vi "DHE_SetSampling.vi"(7 "DBS Ref":T1, 8 "error in":errorcluster, 10 "sampling type":string, 11 "fd":i32) -> (0 "error out":errorcluster, 2 "read value":i32, 3 "fd":i32)   [LabVIEW 2016]
uses:
  DBSHAND/private/vis/DatabaseHand_RefNum.ctl
  DBSHAND/private/vis/DatabaseHand_Element_Set(bool).vi
  DBSHAND/private/vis/DatabaseHand_Element_Set(string).vi
  DBSHAND/private/vis/DatabaseHand_Element_Get(string).vi
  DBSHAND/private/vis/DatabaseHand_Element_Set(I32).vi
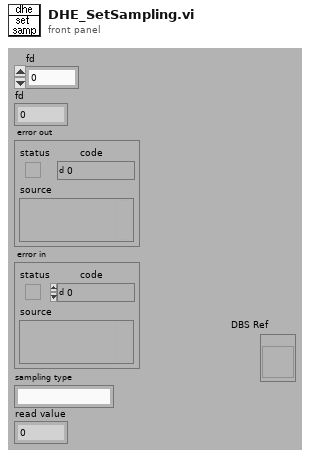
[diagram p1: front panel]
types:
  T1 = typedef "DatabaseHand_RefNum.ctl" = refnum<vi>
  T2 = cluster{"Video Processor Type":string, "support gain":bool, "Timing Board":string, "support reset":bool, "Utility Board":string, "Shutter":string, "Temperature":string, "support temp control":bool, "Detector Type":string, "Support MPP":string, "Support Binning":string, "Readout Mode":string, "support shutter control":bool}
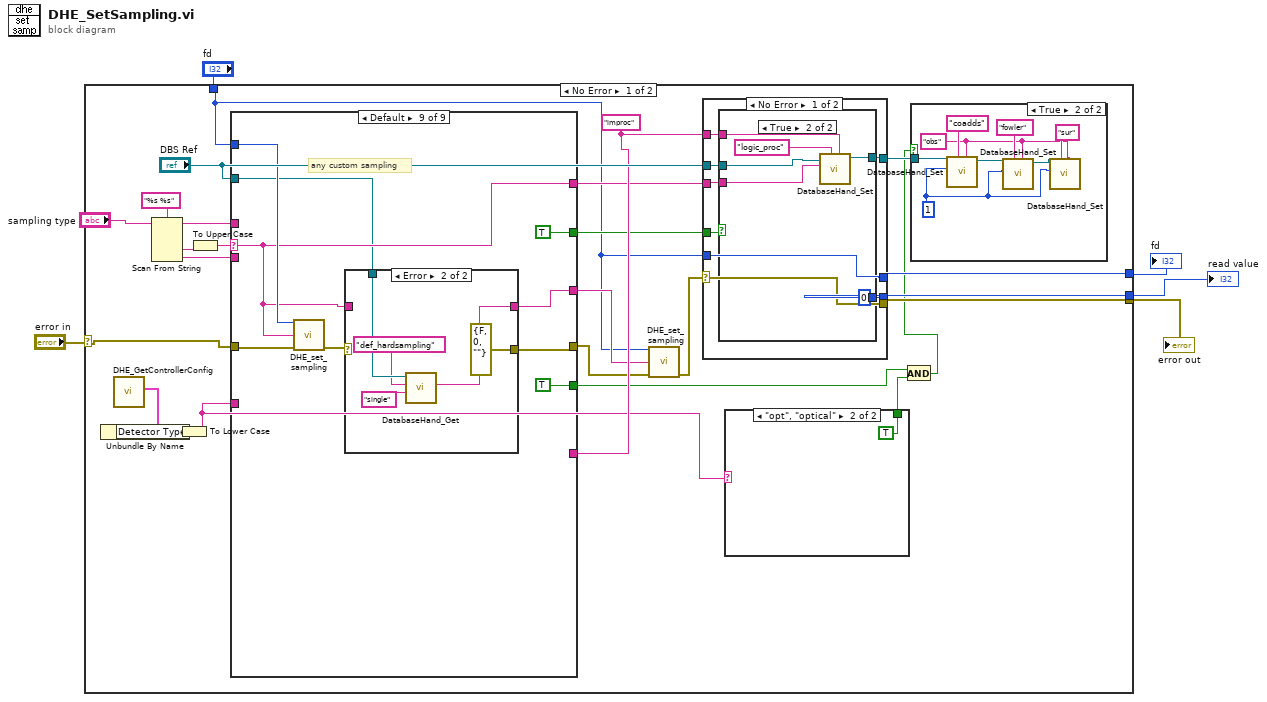
[diagram p0: block diagram]
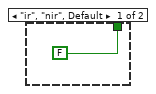
[diagram p2: hidden frame]
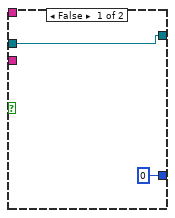
[diagram p4: hidden frame]
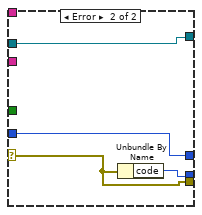
[diagram p5: hidden frame]
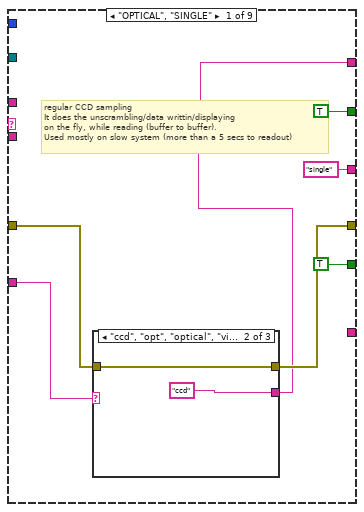
[diagram p6: hidden frame]
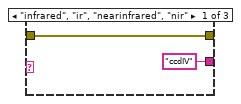
[diagram p7: hidden frame]
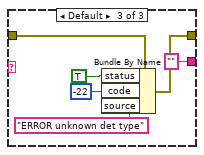
[diagram p8: hidden frame]
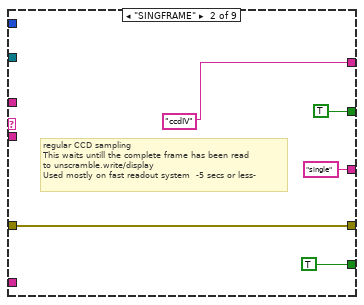
[diagram p9: hidden frame]
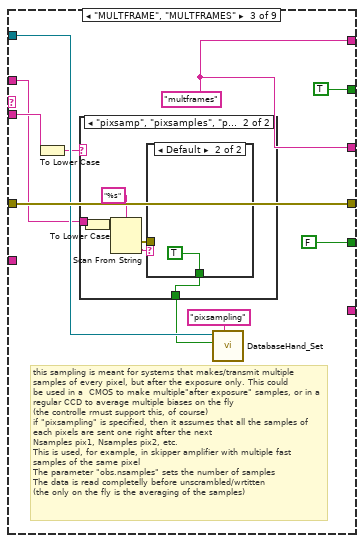
[diagram p10: hidden frame]
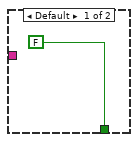
[diagram p11: hidden frame]
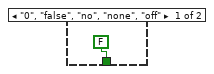
[diagram p12: hidden frame]
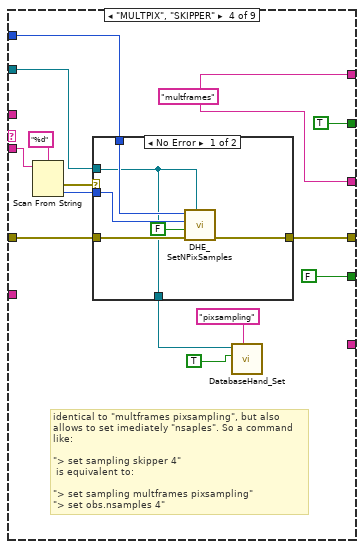
[diagram p13: hidden frame]
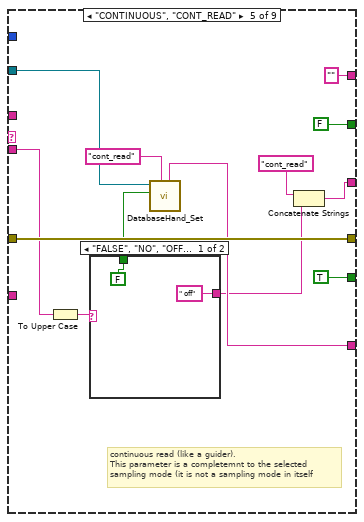
[diagram p15: hidden frame]
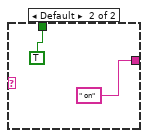
[diagram p16: hidden frame]
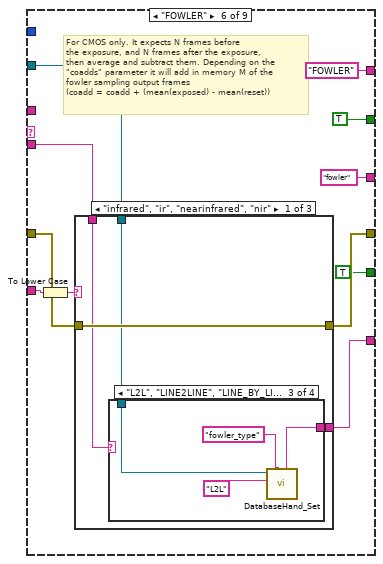
[diagram p17: hidden frame]
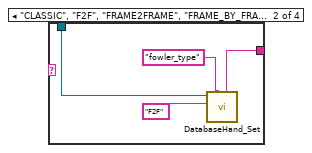
[diagram p19: hidden frame]
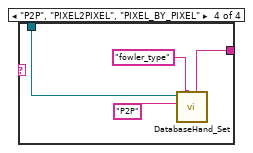
[diagram p20: hidden frame]
diagram:
  n1 = case shown="No Error" "error in" {
    selector: "error in" -> [w23 w243]
    tunnel: [w27 w244] -> w5
    tunnel: [w26 w243] -> w4
    tunnel: [w24 w242] -> w3
    tunnel: "fd" -> [w6 w244]
    frame No Error {
      w19 = "improc" ("group")
      n2 = call "DHE_GetControllerConfig.vi"() -> ("ControllerConfigCluster"=w18:T2)  [unwired: 11 out]
      n3 = Unbundle By Name(w18) -> ("Detector Type"=w13:string)
      n4 = Scan From String(format string="%s %s", input string="sampling type") -> (remaining string=w7:string, output 1=w29:string, output 2=w20:string)  [unwired: 2 in, 4 out]
      n5 = To Lower Case(string=w13) -> (all lower case string=w12:string)
      n6 = To Upper Case(1:w29) -> (0:w28:string)
      n7 = case shown="Default" w28 {
        selector: w28 -> [_ _ _ _ _ _ _ _ w229]
        tunnel: w23 -> [w65 w82 w92 w106 w134 w149 w181 w195 w232]
        tunnel: [w64 w82 w92 w105 w134 w148 w181 w201 w227] -> w16
        tunnel: [w63 "ccdIV" w89 w113 "" "FOWLER" "SUR" "DCS" w229] -> w17
        tunnel: "DBS Ref" -> [_ _ w88 w103 w133 w142 w184 w198 w226]
        tunnel: w20 -> [_ _ w86 w110 w130 w145 w185 w197 _]
        tunnel: w19 -> [_ _ _ _ w132 w144 w183 w196 _]
        tunnel: w12 -> [w66 _ _ _ _ w151 _ w203 _]
        tunnel: ["single" "single" w89 w113 w126 "fowler" "sur" "cds" w228] -> w14
        tunnel: [TRUE TRUE TRUE TRUE FALSE TRUE TRUE TRUE TRUE] -> w11
        tunnel: [TRUE ("x") TRUE ("x") FALSE ("x") FALSE ("x") TRUE ("x") TRUE ("x") TRUE ("x") TRUE ("x") TRUE ("x")] -> w8
        tunnel: w7 -> [_ _ w83 _ _ _ _ _ _]
        tunnel: w6 -> [_ _ _ w104 _ _ _ _ w231]
        frame "OPTICAL", "SINGLE" {
          # "regular CCD sampling\nIt does the unscrambling/data writtin/displaying\non the fly, while reading (buffer to buffer).\nUsed mostly on slow system (more than a 5 secs to readout)"
          n8 = case shown="\"ccd\", \"opt\", \"optical\", \"visible\"" w66 {
            tunnel: ["ccdIV" "ccd" ""] -> w63
            tunnel: w65 -> [w68 w71 w77]
            tunnel: [w68 w71 w76] -> w64
            frame "infrared", "ir", "nearinfrared", "nir" {
            }
            frame "ccd", "opt", "optical", "visible" {
            }
            frame Default {
              n9 = Bundle By Name(cluster=w77, "status"=TRUE, "code"=-22, "source"="ERROR unknown det type") -> (w76:errorcluster)
            }
          }
        }
        frame "SINGFRAME" {
          # "regular CCD sampling\nThis waits untill the complete frame has been read\nto unscramble.write/display\nUsed mostly on fast readout system  -5 secs or less-"
        }
        frame "MULTFRAME", "MULTFRAMES" {
          w89 = "multframes"
          # "this sampling is meant for systems that makes/transmit multiple\nsamples of every pixel, but after the exposure only. This could\nbe used in a  CMOS to make multiple\"after exposure\" samples, or in a regular CCD to average multiple biases on the fly\n(the controlle rmust support this, of course)\nif \"pixsampling\" is specified, then it assumes that all the samples of each pixels are sent one right after the next\nNsamples pix1, Nsamples pix2, etc.\nThis is used, for example, in skipper amplifier with multiple fast samples of the same pixel \nThe parameter \"obs.nsamples\" sets the number of samples\nThe data is read completelly before unscrambled/wrtitten\n(the only on the fly is the averaging of the samples)"
          n10 = To Lower Case(string=w86) -> (all lower case string=w85:string)
          n11 = case shown="\"pixsamp\", \"pixsamples\", \"pixsampling\", \"seqpix\", \"skipper\"" w85 {
            tunnel: [FALSE w95] -> w84
            tunnel: w83 -> [_ w99]
            frame Default {
            }
            frame "pixsamp", "pixsamples", "pixsampling", "seqpix", "skipper" {
              n12 = To Lower Case(string=w99) -> (all lower case string=w96:string)
              n13 = Scan From String(format string="%s", input string=w96) -> (error out=w94:errorcluster, output 1=w97:string)  [unwired: 2 in, 3 out]
              n14 = case shown="Default" w97 {
                tunnel: [FALSE TRUE] -> w95
                tunnel: w94 -> [_ _]
                frame "0", "false", "no", "none", "off" {
                }
                frame Default {
                }
              }
            }
          }
          n15 = call-poly "DatabaseHand_Set.vi"("name"="pixsampling", "value"=w84, "Database RefNum in"=w88) -> ()  [unwired: 5 in, 4 out]
        }
        frame "MULTPIX", "SKIPPER" {
          w113 = "multframes"
          # "identical to \"multframes pixsampling\", but also\nallows to set imediately \"nsaples\". So a command like:\n\n\"> set sampling skipper 4\"\n is equivalent to:\n\n\"> set sampling multframes pixsampling\"\n\"> set obs.nsamples 4\""
          n16 = Scan From String(format string="%d", input string=w110) -> (error out=w108:errorcluster, output 1=w107:i32)  [unwired: 2 in, 3 out]
          n17 = case shown="No Error" w108 {
            tunnel: w107 -> [w119 _]
            tunnel: w106 -> [w121 w123]
            tunnel: [w120 w123] -> w105
            tunnel: w104 -> [w118 _]
            tunnel: w103 -> [w117 w122]
            tunnel: [w117 w122] -> w102
            frame No Error {
              n18 = call "DHE_SetNPixSamples.vi"("Database RefNum in"=w117, "error in (no error)"=w121, "check sampling"=FALSE, "nsamples"=w119, "fd"=w118) -> ("error IO"=w120:errorcluster)  [unwired: 6 out]
            }
            frame Error {
            }
          }
          n19 = call-poly "DatabaseHand_Set.vi"("name"="pixsampling", "value"=TRUE, "Database RefNum in"=w102) -> ()  [unwired: 5 in, 4 out]
        }
        frame "CONTINUOUS", "CONT_READ" {
          # "continuous read (like a guider).\nThis parameter is a completemnt to the selected\nsampling mode (it is not a sampling mode in itself"
          n20 = To Upper Case(1:w130) -> (0:w129:string)
          n21 = case shown="\"FALSE\", \"NO\", \"OFF\"" w129 {
            tunnel: [FALSE TRUE] -> w128
            tunnel: [" off" " on"] -> w125
            frame "FALSE", "NO", "OFF" {
            }
            frame Default {
            }
          }
          n22 = call-poly "DatabaseHand_Set.vi"("group"=w132, "name"="cont_read", "value"=w128, "Database RefNum in"=w133) -> ()  [unwired: 4 in, 4 out]
          n23 = Concatenate Strings("cont_read", w125) -> (w126:string)
        }
        frame "FOWLER" {
          # "For CMOS only. It expects N frames before\nthe exposure, and N frames after the exposure,\nthen average and subtract them. Depending on the\n\"coadds\" parameter it will add in memory M of the\nfowler sampling output frames\n(coadd = coadd + (mean(exposed) - mean(reset))"
          n24 = To Lower Case(string=w151) -> (all lower case string=w150:string)
          n25 = case shown="\"infrared\", \"ir\", \"nearinfrared\", \"nir\"" w150 {
            tunnel: w149 -> [w155 w172 w177]
            tunnel: [w155 w171 w176] -> w148
            tunnel: w145 -> [w154 _ _]
            tunnel: w144 -> [w153 _ _]
            tunnel: w142 -> [w152 _ _]
            frame "infrared", "ir", "nearinfrared", "nir" {
              n26 = case shown="\"L2L\", \"LINE2LINE\", \"LINE_BY_LINE\"" w154 {
                tunnel: w153 -> [_ w158 w162 w166]
                tunnel: w152 -> [_ w156 w160 w164]
                frame Default {
                }
                frame "CLASSIC", "F2F", "FRAME2FRAME", "FRAME_BY_FRAME", "NORMAL" {
                  n27 = call-poly "DatabaseHand_Set.vi"("group"=w158, "name"="fowler_type", "value"="F2F", "Database RefNum in"=w156) -> ()  [unwired: 4 in, 4 out]
                }
                frame "L2L", "LINE2LINE", "LINE_BY_LINE" {
                  n28 = call-poly "DatabaseHand_Set.vi"("group"=w162, "name"="fowler_type", "value"="L2L", "Database RefNum in"=w160) -> ()  [unwired: 4 in, 4 out]
                }
                frame "P2P", "PIXEL2PIXEL", "PIXEL_BY_PIXEL" {
                  n29 = call-poly "DatabaseHand_Set.vi"("group"=w166, "name"="fowler_type", "value"="P2P", "Database RefNum in"=w164) -> ()  [unwired: 4 in, 4 out]
                }
              }
            }
            frame "ccd", "opt", "optical", "visible" {
              n30 = Bundle By Name(cluster=w172, "status"=TRUE, "code"=-1, "source"="ERROR unsupported") -> (w171:errorcluster)
            }
            frame Default {
              (unwired) ""
              n31 = Bundle By Name(cluster=w177, "status"=TRUE, "code"=-22, "source"="ERROR unknown det type") -> (w176:errorcluster)
            }
          }
        }
        frame "SUR" {
          # "Sample Up The Ramp. \nCMOS only. It expect 1 frame before the exposure and\nN frames after, and writes them all down to disk with\nno processing"
          n32 = case shown="Default" w185 {
            tunnel: w184 -> [_ w186 w190]
            tunnel: w183 -> [_ _ w189]
            frame Default {
            }
            frame "NORMALIZED" {
              n33 = call-poly "DatabaseHand_Set.vi"("name"="normalize_sur", "value"=TRUE, "Database RefNum in"=w186) -> ()  [unwired: 5 in, 4 out]
            }
            frame "RAW" {
              n34 = call-poly "DatabaseHand_Set.vi"("group"=w189, "name"="normalize_sur", "value"=FALSE, "Database RefNum in"=w190) -> ()  [unwired: 4 in, 4 out]
            }
          }
        }
        frame "CDS", "DCS" {
          # "CMOS only. It does a clasical Correlated Double Sampling\non the reset (befor eexposure) and the exposed\n(after exposure) frames.\nThis is equivalent to FOWLER sampling with \nnsamples=1"
          n35 = To Lower Case(string=w203) -> (all lower case string=w202:string)
          n36 = case shown="\"ccd\", \"opt\", \"optical\", \"visible\"" w202 {
            tunnel: w195 -> [w204 w220 w225]
            tunnel: [w204 w219 w224] -> w201
            tunnel: w198 -> [w207 _ _]
            tunnel: w197 -> [w206 _ _]
            tunnel: w196 -> [w205 _ _]
            frame "infrared", "ir", "nearinfrared", "nir" {
              n37 = case shown="\"NORMAL\"" w206 {
                tunnel: w207 -> [_ w211 w215]
                tunnel: w205 -> [_ w208 w212]
                frame Default {
                }
                frame "INVERSE" {
                  n38 = call-poly "DatabaseHand_Set.vi"("group"=w208, "name"="inversecds", "value"=TRUE, "Database RefNum in"=w211) -> ()  [unwired: 4 in, 4 out]
                }
                frame "NORMAL" {
                  n39 = call-poly "DatabaseHand_Set.vi"("group"=w212, "name"="inversecds", "value"=FALSE, "Database RefNum in"=w215) -> ()  [unwired: 4 in, 4 out]
                }
              }
            }
            frame "ccd", "opt", "optical", "visible" {
              n40 = Bundle By Name(cluster=w220, "status"=TRUE, "code"=-1, "source"="ERROR unsupported") -> (w219:errorcluster)
            }
            frame Default {
              n41 = Bundle By Name(cluster=w225, "status"=TRUE, "code"=-22, "source"="ERROR unknown det type") -> (w224:errorcluster)
            }
          }
        }
        frame Default {
          # "any custom sampling"
          n42 = call "DHE_set_sampling.vi"("fd"=w231, "sampling"=w229, "error in (no error)"=w232) -> ("error out"=w230:errorcluster)  [unwired: 12 out]
          n43 = case shown="Error" w230 {
            selector: w230 -> [w235 _]
            tunnel: w229 -> [w236 _]
            tunnel: [w236 w238] -> w228
            tunnel: [w235 errorcluster {"status"=FALSE, "code"=0, "source"=""} ("error IO")] -> w227
            tunnel: w226 -> [_ w241]
            frame No Error {
            }
            frame Error {
              n44 = call-poly "DatabaseHand_Get.vi"("default value"="single", "name"="def_hardsampling", "Database RefNum in"=w241) -> ("value"=w238:string)  [unwired: 2 in, 6 out]
            }
          }
        }
      }
      n45 = call "DHE_set_sampling.vi"("fd"=w6, "sampling"=w14, "error in (no error)"=w16) -> ("error out"=w15:errorcluster)  [unwired: 12 out]
      n46 = case shown="No Error" w15 {
        selector: w15 -> [w46 w59]
        tunnel: w6 -> [w47 w60]
        tunnel: [w47 w60] -> w27
        tunnel: [w45 w58] -> w24
        tunnel: [w46 w59] -> w26
        tunnel: w19 -> [w44 _]
        tunnel: "DBS Ref" -> [w48 w57]
        tunnel: w17 -> [w42 _]
        tunnel: [w43 w57] -> w22
        tunnel: w11 -> [w41 _]
        frame No Error {
          n47 = case shown="True" w41 {
            tunnel: w48 -> [w50 w55]
            tunnel: [0 ("code") 0 ("code")] -> w45
            tunnel: w44 -> [_ w53]
            tunnel: [w50 w52] -> w43
            tunnel: w42 -> [_ w51]
            frame False {
            }
            frame True {
              n48 = call-poly "DatabaseHand_Set.vi"("group"=w53, "name"="logic_proc", "value"=w51, "Database RefNum in"=w55) -> ("Database RefNum out"=w52:T1)  [unwired: 4 in, 3 out]
            }
          }
        }
        frame Error {
          n49 = Unbundle By Name(w59) -> ("code"=w58:i32)
        }
      }
      n50 = case shown="\"opt\", \"optical\"" w12 {
        tunnel: [FALSE TRUE] -> w10
        frame "ir", "nir", Default {
        }
        frame "opt", "optical" {
        }
      }
      n51 = And(x=w8, y=w10) -> (x .and. y?=w9:bool)
      n52 = case shown="True" w9 {
        tunnel: w22 -> [_ w40]
        frame False {
        }
        frame True {
          w33 = "obs" ("group")
          w34 = 1
          n53 = call-poly "DatabaseHand_Set.vi"("group"=w33, "name"="coadds", "value"=w34, "Database RefNum in"=w40) -> ("Database RefNum out"=w39:T1)  [unwired: 4 in, 3 out]
          n54 = call-poly "DatabaseHand_Set.vi"("group"=w33, "name"="fowler", "value"=w34, "Database RefNum in"=w39) -> ("Database RefNum out"=w38:T1)  [unwired: 4 in, 3 out]
          n55 = call-poly "DatabaseHand_Set.vi"("group"=w33, "name"="sur", "value"=w34, "Database RefNum in"=w38) -> ()  [unwired: 4 in, 4 out]
        }
      }
    }
    frame Error {
      n56 = Unbundle By Name(w243) -> ("code"=w242:i32)
    }
  }
  "fd" <- w5
  "error out" <- w4
  "read value" <- w3
